vi "2D String Array to String.vi"(6 "Delimiter (,)":string=",", 11 "2D Array[]":string[][](array[string])) -> (3 "String":string)   [LabVIEW 2016, in "SLL String.lvlib"]
uses:
  SLL String.lvlib
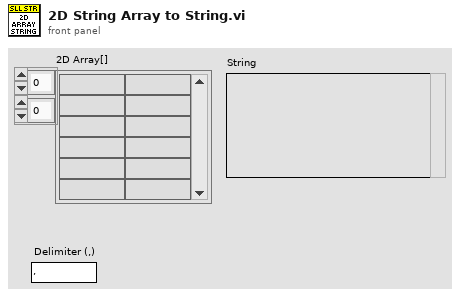
[diagram p1: front panel]
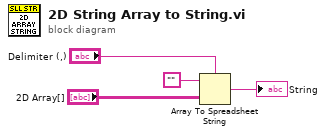
[diagram p0: block diagram]
diagram:
  n1 = Array To Spreadsheet String(delimiter (Tab)="Delimiter (,)", array="2D Array[]", 3:"") -> (spreadsheet string=→"String":string)
